vi "getPositionsAndVoltages.vi"(0 "connection ID":i32, 5 "error in":errorcluster) -> (14 "connection ID":i32, 19 "error out":errorcluster)   [LabVIEW 2016]
doc: "Simultaneously get 3 axes positions as well as the DC offset\n to maximize sampling rate over network"
panel:
  out "val3":i32
  out "val2":i32
  out "val1":i32
  out "pos3":i32
  out "pos2":i32
  out "pos1":i32
  out "params_cluster":cluster{"Numeric":i32}
  in  "Params_cluster":cluster{"Numeric":dbl}
  in  "results_cluster":T1
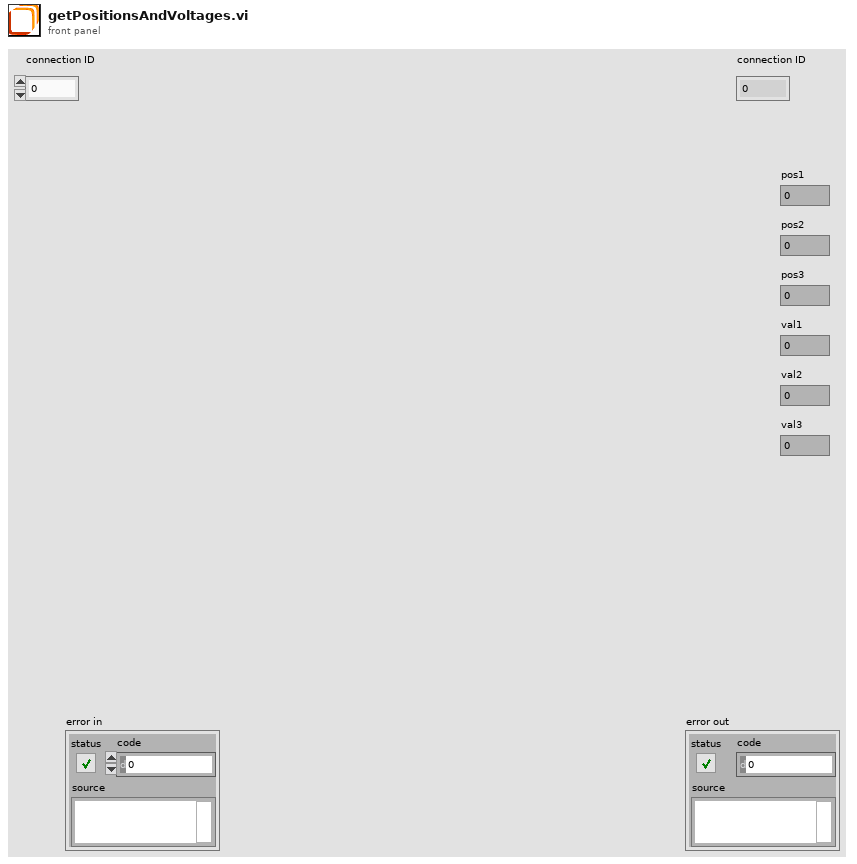
[diagram p1: front panel]
types:
  T1 = cluster{"errNo":i32, "pos1":i32, "pos2":i32, "pos3":i32, "val1":i32, "val2":i32, "val3":i32}
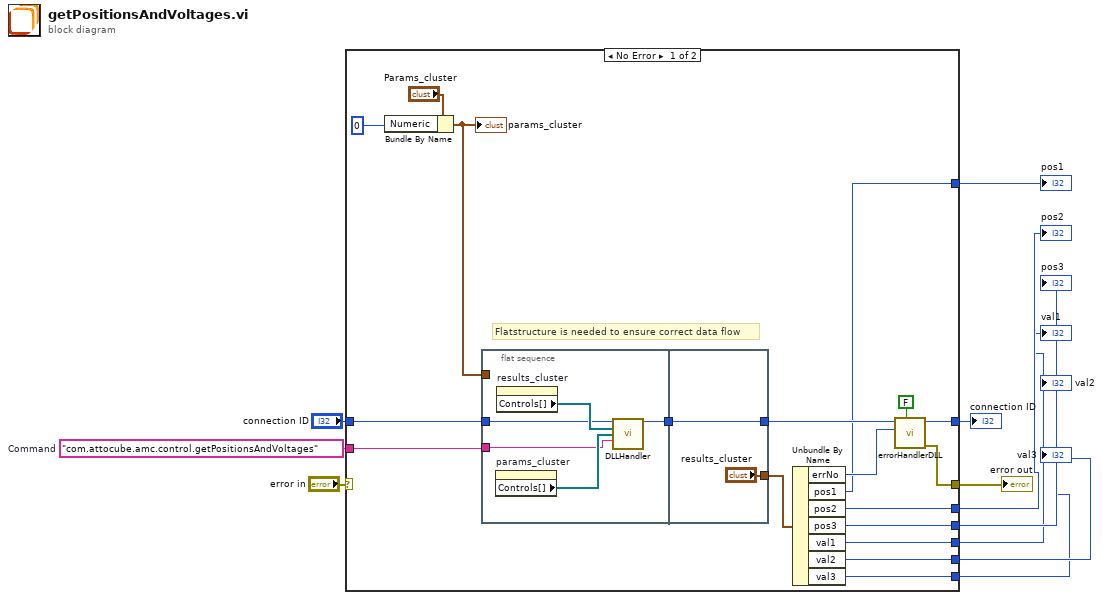
[diagram p0: block diagram]
diagram:
  w9 = "com.attocube.amc.control.getPositionsAndVoltages"  # Command
  n1 = case shown="No Error" "error in" {
    selector: "error in" -> [_ w38]
    tunnel: [w28 w38] -> w11
    tunnel: w9 -> [w23 _]
    tunnel: [w22 w37] -> w8
    tunnel: "connection ID" -> [w21 w37]
    tunnel: [w17 _] -> w6
    tunnel: [w16 _] -> w5
    tunnel: [w15 _] -> w4
    tunnel: [w14 _] -> w3
    tunnel: [w13 _] -> w2
    tunnel: [w12 _] -> w1
    frame No Error {
      # "Flatstructure is needed to ensure correct data flow"
      n2 = Bundle By Name(cluster="Params_cluster", "Numeric"=0) -> (w19:cluster{"Numeric":dbl})
      "params_cluster" <- w19
      n3 = flat-sequence {
        tunnel: [w34] -> w25
        tunnel: w23 -> [w31]
        tunnel: w21 -> [w30]
        tunnel: w19 -> [_]
        tunnel: ["results_cluster"] -> w26
        tunnel: [w36] -> w27
        tunnel: w25 -> [w36]
        frame #0 {
          n4 = property on="params_cluster" class="Clust (strict)"() -> ("Controls[]"=w32:refnum<vi>[])  [unwired: 2 in, 2 out]
          n5 = property on="results_cluster" class="Clust (strict)"() -> ("Controls[]"=w33:refnum<vi>[])  [unwired: 2 in, 2 out]
          n6 = call "DLLHandler.vi"("connection ID"=w30, "results_cluster"=w33, "params_cluster"=w32, "method"=w31) -> ("connection ID out"=w34:i32)  [unwired: 10 in, 1 out]
        }
        frame #1 {
        }
      }
      n7 = Unbundle By Name(w26) -> ("errNo"=w20:i32, "pos1"=w17:i32, "pos2"=w16:i32, "pos3"=w15:i32, "val1"=w14:i32, "val2"=w13:i32, "val3"=w12:i32)
      n8 = call "errorHandlerDLL.vi"("show popup"=FALSE, "error number"=w20, "connection ID"=w27) -> ("error out"=w28:errorcluster, "connection ID"=w22:i32)  [unwired: 7 in]
    }
    frame Error {
    }
  }
  "error out" <- w11
  "connection ID" <- w8
  "pos1" <- w6
  "pos2" <- w5
  "pos3" <- w4
  "val1" <- w3
  "val2" <- w2
  "val3" <- w1
